vi "AlgorithmLeftGoal.vi"(6 "MatchBallY":dbl, 7 "MatchBallX":dbl, 8 "D2 Y COM":dbl, 9 "D2 X COM":dbl, 10 "D1Y COM":dbl, 11 "D1 X COM":dbl) -> (0 "min x3":dbl, 1 "aS":dbl, 2 "min x2":dbl, 3 "aRW":dbl, 4 "min x":dbl, 5 "Theta LG,LW":dbl)   [LabVIEW 2014]
panel:
  out "output cluster":cluster{"m":dbl, "y":dbl, "y":dbl}
  out "RW":cluster{"kRW":dbl, "CoRW":dbl, "y":dbl}
  out "LW":cluster{"kLW":dbl, "CoLW":dbl, "y":dbl}
  out "xD2BotS":dbl
  out "xD2ComS":dbl
  out "xD1BotS":dbl
  out "xD1ComS":dbl
  out "xD2BotR":dbl
  out "xD2ComR":dbl
  out "xD1BotR":dbl
  out "xD1ComR":dbl
  out "D2 X Bot fit 2":dbl
  out "D2 X Com fit":dbl
  out "D1 X Bot fit":dbl
  out "D1 X Com fit":dbl
  # "LOGIC"
  # "Left Goal"
  # "STRAIGHT"
  # "Left wall"
  # "Right Wall"
  # "Straight"
  # "sending data"
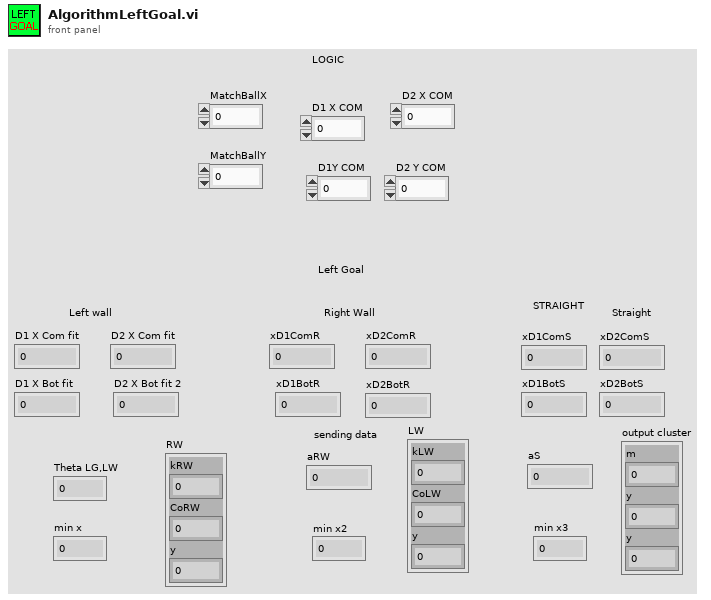
[diagram p1: front panel]
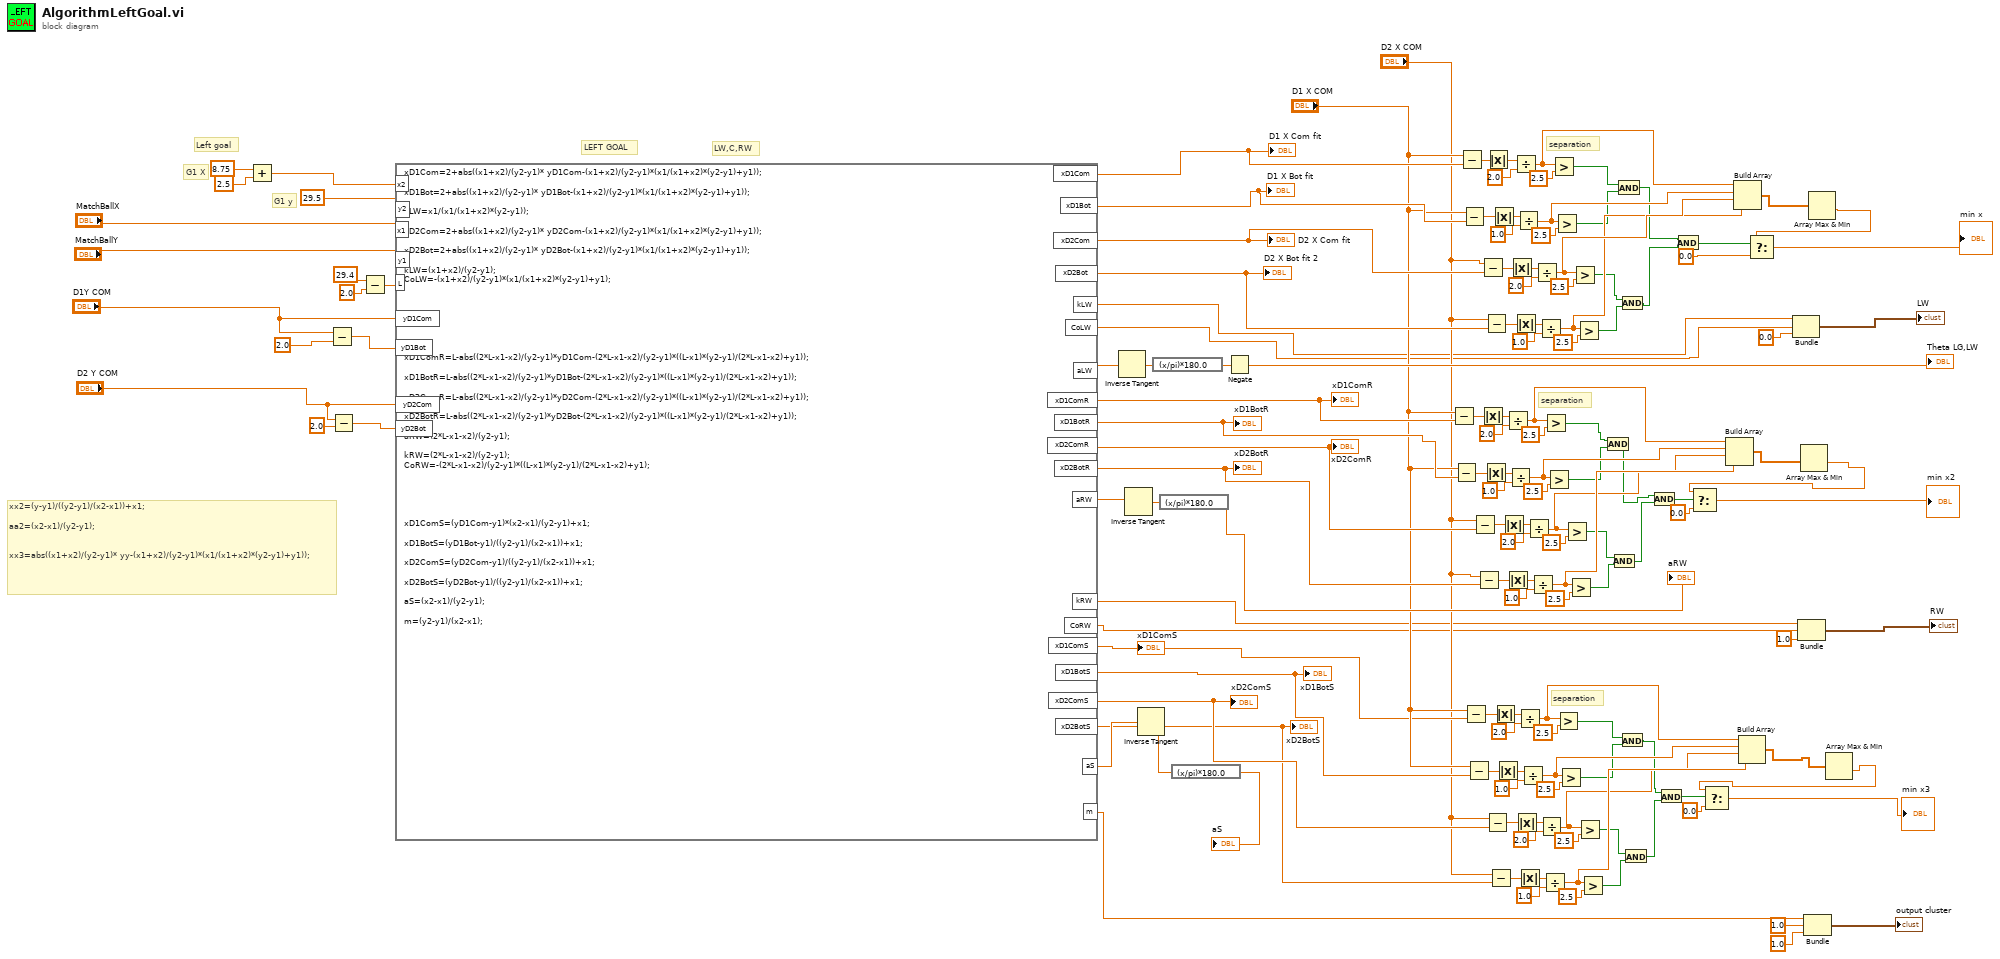
[diagram p0: block diagram]
diagram:
  # "LW,C,RW"
  # "separation"
  # "separation"
  # "separation"
  # "LEFT GOAL"
  # "xx2=(y-y1)/((y2-y1)/(x2-x1))+x1;\n\naa2=(x2-x1)/(y2-y1);\n\n\nxx3=abs((x1+x2)/(y2-y1)* yy-(x1+x2)/(y2-y1)*(x1/(x1+x2)*(y2-y1)+y1));"
  # "Left goal"
  # "G1 y"
  # "G1 X"
  n1 = Add(x=8.75, y=2.5) -> (x+y=w139:dbl)
  n2 = Subtract(x="D1Y COM", y=2.0) -> (x-y=w134:dbl)
  n3 = Subtract(x="D2 Y COM", y=2.0) -> (x-y=w129:dbl)
  n4 = Subtract(x=29.4 ("input variable"), y=2.0) -> (x-y=w14:dbl)
  n5 = formula code="xD1Com=2+abs((x1+x2)/(y2-y1)* yD1Com-(x1+x2)/(y2-y1)*(x1/(x1+x2)*(y2-y1)+y1));\n\nxD1Bot=2+abs((x1+x2)/(y2-y1)* yD1Bot-(x1+x2)/(y2-y1)*(x1/(x1+x2)*(y2-y1)+y1));\n\naLW=x1/(x1/(x1+x2)*(y2-y1));\n\nxD2Com=2+abs((x1+x2)/(y2-y1)* yD2Com-(x1+x2)/(y2-y1)*(x1/(x1+x2)*(y2-y1)+y1));\n\nxD2Bot=2+abs((x1+x2)/(y2-y1)* yD2Bot-(x1+x2)/(y2-y1)*(x1/(x1+x2)*(y2-y1)+y1));\n\nkLW=(x1+x2)/(y2-y1);\nCoLW=-(x1+x2)/(y2-y1)*(x1/(x1+x2)*(y2-y1)+y1);\n\n\n\n\n\n\n\nxD1ComR=L-abs((2*L-x1-x2)/(y2-y1)*yD1Com-(2*L-x1-x2)/(y2-y1)*((L-x1)*(y2-y1)/(2*L-x1-x2)+y1));\n\nxD1BotR=L-abs((2*L-x1-x2)/(y2-y1)*yD1Bot-(2*L-x1-x2)/(y2-y1)*((L-x1)*(y2-y1)/(2*L-x1-x2)+y1));\n\nxD2ComR=L-abs((2*L-x1-x2)/(y2-y1)*yD2Com-(2*L-x1-x2)/(y2-y1)*((L-x1)*(y2-y1)/(2*L-x1-x2)+y1));\n\nxD2BotR=L-abs((2*L-x1-x2)/(y2-y1)*yD2Bot-(2*L-x1-x2)/(y2-y1)*((L-x1)*(y2-y1)/(2*L-x1-x2)+y1));\n\naRW=(2*L-x1-x2)/(y2-y1);\n\nkRW=(2*L-x1-x2)/(y2-y1);\nCoRW=-(2*L-x1-x2)/(y2-y1)*((L-x1)*(y2-y1)/(2*L-x1-x2)+y1);\n\n\n\n\n\nxD1ComS=(yD1Com-y1)*(x2-x1)/(y2-y1)+x1;\n\nxD1BotS=(yD1Bot-y1)/((y2-y1)/(x2-x1))+x1;\n\nxD2ComS=(yD2Com-y1)/((y2-y1)/(x2-x1))+x1;\n\nxD2BotS=(yD2Bot-y1)/((y2-y1)/(x2-x1))+x1;\n\naS=(x2-x1)/(y2-y1);\n\nm=(y2-y1)/(x2-x1);"("x1"="MatchBallX", "x2"=w139, "y2"=29.5, "y1"="MatchBallY", "yD1Com"="D1Y COM", "yD2Com"="D2 Y COM", "yD1Bot"=w134, "yD2Bot"=w129, "L"=w14) -> ("xD1Com"=w122:dbl, "aLW"=w137:dbl, "xD1Bot"=w108:dbl, "xD2Com"=w113:dbl, "xD2Bot"=w103:dbl, "xD1ComR"=w76:dbl, "xD1BotR"=w75:dbl, "xD2ComR"=w74:dbl, "xD2BotR"=w73:dbl, "aRW"=w127:dbl, "xD1ComS"=w50:dbl, "aS"=w123:dbl, "xD1BotS"=w49:dbl, "xD2BotS"=w47:dbl, "xD2ComS"=w48:dbl, "kLW"=w12:dbl, "CoLW"=w11:dbl, "kRW"=w8:dbl, "CoRW"=w7:dbl, "m"=w4:dbl)
  "D1 X Com fit" <- w122
  "D1 X Bot fit" <- w108
  "D2 X Com fit" <- w113
  "D2 X Bot fit 2" <- w103
  "xD1ComR" <- w76
  "xD1BotR" <- w75
  "xD2ComR" <- w74
  "xD2BotR" <- w73
  "xD1ComS" <- w50
  "xD1BotS" <- w49
  "xD2ComS" <- w48
  "xD2BotS" <- w47
  n6 = Inverse Tangent(1:w137) -> (0:w138:dbl)
  n7 = Inverse Tangent(1:w127) -> (0:w128:dbl)
  n8 = Inverse Tangent(1:w123) -> (0:w124:dbl)
  n9 = expression code="(x/pi)*180.0" ("radians to degrees")(w138) -> (w135:dbl)
  n10 = expression code="(x/pi)*180.0" ("radians to degrees")(w128) -> (→"aRW":dbl)
  n11 = expression code="(x/pi)*180.0" ("radians to degrees")(w124) -> (→"aS":dbl)
  n12 = Negate(x=w135) -> (-x=→"Theta LG,LW":dbl)
  n13 = Subtract(x="D1 X COM", y=w76) -> (x-y=w77:dbl)
  n14 = Subtract(x="D1 X COM", y=w75) -> (x-y=w88:dbl)
  n15 = Subtract(x="D1 X COM", y=w122) -> (x-y=w121:dbl)
  n16 = Subtract(x="D1 X COM", y=w108) -> (x-y=w109:dbl)
  n17 = Subtract(x="D1 X COM", y=w50) -> (x-y=w52:dbl)
  n18 = Subtract(x="D1 X COM", y=w49) -> (x-y=w63:dbl)
  n19 = Subtract(x="D2 X COM", y=w74) -> (x-y=w84:dbl)
  n20 = Subtract(x="D2 X COM", y=w73) -> (x-y=w89:dbl)
  n21 = Subtract(x="D2 X COM", y=w113) -> (x-y=w114:dbl)
  n22 = Absolute Value(x=w77) -> (abs(x)=w78:dbl)
  n23 = Absolute Value(x=w88) -> (abs(x)=w87:dbl)
  n24 = Subtract(x="D2 X COM", y=w103) -> (x-y=w107:dbl)
  n25 = Subtract(x="D2 X COM", y=w48) -> (x-y=w59:dbl)
  n26 = Absolute Value(x=w121) -> (abs(x)=w120:dbl)
  n27 = Subtract(x="D2 X COM", y=w47) -> (x-y=w64:dbl)
  n28 = Absolute Value(x=w109) -> (abs(x)=w110:dbl)
  n29 = Absolute Value(x=w52) -> (abs(x)=w53:dbl)
  n30 = Absolute Value(x=w63) -> (abs(x)=w62:dbl)
  n31 = Absolute Value(x=w84) -> (abs(x)=w83:dbl)
  n32 = Divide(x=w78, y=2.0) -> (x/y=w94:dbl)
  n33 = Absolute Value(x=w89) -> (abs(x)=w90:dbl)
  n34 = Divide(x=w87, y=1.0) -> (x/y=w95:dbl)
  n35 = Absolute Value(x=w114) -> (abs(x)=w115:dbl)
  n36 = Divide(x=w120, y=2.0) -> (x/y=w101:dbl)
  n37 = Absolute Value(x=w107) -> (abs(x)=w106:dbl)
  n38 = Absolute Value(x=w59) -> (abs(x)=w58:dbl)
  n39 = Divide(x=w110, y=1.0) -> (x/y=w100:dbl)
  n40 = Divide(x=w53, y=2.0) -> (x/y=w69:dbl)
  n41 = Absolute Value(x=w64) -> (abs(x)=w65:dbl)
  n42 = Divide(x=w62, y=1.0) -> (x/y=w70:dbl)
  n43 = Divide(x=w83, y=2.0) -> (x/y=w96:dbl)
  n44 = Divide(x=w90, y=1.0) -> (x/y=w97:dbl)
  n45 = Divide(x=w115, y=2.0) -> (x/y=w99:dbl)
  n46 = Divide(x=w106, y=1.0) -> (x/y=w98:dbl)
  n47 = Divide(x=w58, y=2.0) -> (x/y=w71:dbl)
  n48 = Divide(x=w65, y=1.0) -> (x/y=w72:dbl)
  n49 = Greater?(x=w94, y=2.5) -> (0:w33:bool)
  n50 = Greater?(x=w95, y=2.5) -> (0:w32:bool)
  n51 = Greater?(x=w101, y=2.5) -> (0:w38:bool)
  n52 = Greater?(x=w100, y=2.5) -> (0:w37:bool)
  n53 = Greater?(x=w69, y=2.5) -> (0:w28:bool)
  n54 = Greater?(x=w70, y=2.5) -> (0:w27:bool)
  n55 = Greater?(x=w96, y=2.5) -> (0:w31:bool)
  n56 = Greater?(x=w97, y=2.5) -> (0:w30:bool)
  n57 = Greater?(x=w99, y=2.5) -> (0:w42:bool)
  n58 = Greater?(x=w98, y=2.5) -> (0:w41:bool)
  n59 = Greater?(x=w71, y=2.5) -> (0:w25:bool)
  n60 = Greater?(x=w72, y=2.5) -> (0:w24:bool)
  n61 = And(x=w33, y=w32) -> (x .and. y?=w34:bool)
  n62 = And(x=w31, y=w30) -> (x .and. y?=w29:bool)
  n63 = And(x=w38, y=w37) -> (x .and. y?=w36:bool)
  n64 = And(x=w42, y=w41) -> (x .and. y?=w39:bool)
  n65 = And(x=w28, y=w27) -> (x .and. y?=w26:bool)
  n66 = And(x=w25, y=w24) -> (x .and. y?=w23:bool)
  n67 = And(x=w34, y=w29) -> (x .and. y?=w35:bool)
  n68 = And(x=w26, y=w23) -> (x .and. y?=w22:bool)
  n69 = And(x=w36, y=w39) -> (x .and. y?=w40:bool)
  n70 = Build Array(w94, w95, w96, w97) -> (w19:dbl[])
  n71 = Build Array(w101, w100, w99, w98) -> (w21:dbl[])
  n72 = Build Array(w69, w70, w71, w72) -> (w17:dbl[])
  n73 = Bundle("kLW"=w12, "CoLW"=w11, "y"=0.0) -> (→"LW":cluster{"kLW":dbl, "CoLW":dbl, "y":dbl})  [unwired: 1 in]
  n74 = Bundle("kRW"=w8, "CoRW"=w7, "y"=1.0) -> (→"RW":cluster{"kRW":dbl, "CoRW":dbl, "y":dbl})  [unwired: 1 in]
  n75 = Array Max & Min(array=w19) -> (min value=w18:dbl)  [unwired: 3 out]
  n76 = Select(t=w18, s=w35, f=0.0 ("y")) -> (s? t:f=→"min x2":dbl)
  n77 = Bundle("m"=w4, "y"=1.0, "y"=1.0) -> (→"output cluster":cluster{"m":dbl, "y":dbl, "y":dbl})  [unwired: 1 in]
  n78 = Array Max & Min(array=w21) -> (min value=w20:dbl)  [unwired: 3 out]
  n79 = Select(t=w20, s=w40, f=0.0 ("y")) -> (s? t:f=→"min x":dbl)
  n80 = Array Max & Min(array=w17) -> (min value=w16:dbl)  [unwired: 3 out]
  n81 = Select(t=w16, s=w22, f=0.0 ("y")) -> (s? t:f=→"min x3":dbl)
